vi "SVFA Unit Conversion (XY) (N Ch - M Orders).vi"(0 "magnitudes":T1(array[cluster]) {"magnitude" format="%.2f"; "time/rev/rpm" format="%.2f"}, 1 "desired scaling":T8 {"dB reference (0: no change)" format="%.2f"}, 4 "magnitudes info in":T2[](array[typedef]) {"x-axis units" items=["Time (s)"=0, "Frequency-CB (Hz)"=1, "Frequency-CPB (Hz)"=1248, "Frequency-Arbitrary (Hz)"=2357, "Quefrency (s)"=2, "Revolutions (rev)"=3, "Order"=4, "Speed (RPM)"=11, "Speed (rad/s)"=21, "Index"=65535]; "weighting filter" items=["Linear", "A-weighting", "B-weighting", "C-weighting", "ITU-R 468-4", "Dolby", "CCITT", "C-message", "Wb", "Wc", "Wd", "We", "Wf", "Wh", "Wj", "Wk", "Wm", "AES17 20 kHz lowpass", "AES17 40 kHz lowpass", "AES17 20 kHz highpass", "AES17 40 kHz highpass"]; "dB reference [EU]" format="%.2f"; "engineering units" items=["custom..."=0, "V"=1, "A"=21, "C"=30, "pC"=31, "s"=32, "-"=29, "Pa"=2, "N"=20, "g"=3, "m/s^2"=4, "m/s"=5, "m"=6, "mm/s"=12, "mm"=13, "micron/s"=14, "micron"=15, "in/s^2"=7, "in/s"=8, "in"=9, "mil/s"=10, "mil"=11, "rad/s^2"=16, "rad/s"=17, "rad"=18, "deg/s^2"=26, "deg/s"=27, "deg"=28, "RPM"=22, "cycle/s^2"=23, "Hz"=24, "cycle"=25, "strain"=19]; "spectral info"."window" items=["None "=0, "Hanning"=1, "Hamming"=2, "Blackman-Harris"=3, "Exact Blackman"=4, "Blackman"=5, "Flat Top"=6, "4 Term B-Harris "=7, "7 Term B-Harris"=8, "Low Sidelobe"=9, "Force - Exponential"=10, "Gaussian"=62]}, 5 "error in (no error)":errorcluster) -> (14 "converted magnitudes":T1(array[cluster]) {"magnitude" format="%.2f"; "time/rev/rpm" format="%.2f"}, 15 "unit labels":string[](array[string]), 18 "magnitudes info out":T2[](array[typedef]) {"x-axis units" items=["Time (s)"=0, "Frequency-CB (Hz)"=1, "Frequency-CPB (Hz)"=1248, "Frequency-Arbitrary (Hz)"=2357, "Quefrency (s)"=2, "Revolutions (rev)"=3, "Order"=4, "Speed (RPM)"=11, "Speed (rad/s)"=21, "Index"=65535]; "weighting filter" items=["Linear", "A-weighting", "B-weighting", "C-weighting", "ITU-R 468-4", "Dolby", "CCITT", "C-message", "Wb", "Wc", "Wd", "We", "Wf", "Wh", "Wj", "Wk", "Wm", "AES17 20 kHz lowpass", "AES17 40 kHz lowpass", "AES17 20 kHz highpass", "AES17 40 kHz highpass"]; "dB reference [EU]" format="%.2f"; "engineering units" items=["custom..."=0, "V"=1, "A"=21, "C"=30, "pC"=31, "s"=32, "-"=29, "Pa"=2, "N"=20, "g"=3, "m/s^2"=4, "m/s"=5, "m"=6, "mm/s"=12, "mm"=13, "micron/s"=14, "micron"=15, "in/s^2"=7, "in/s"=8, "in"=9, "mil/s"=10, "mil"=11, "rad/s^2"=16, "rad/s"=17, "rad"=18, "deg/s^2"=26, "deg/s"=27, "deg"=28, "RPM"=22, "cycle/s^2"=23, "Hz"=24, "cycle"=25, "strain"=19]; "spectral info"."window" items=["None "=0, "Hanning"=1, "Hamming"=2, "Blackman-Harris"=3, "Exact Blackman"=4, "Blackman"=5, "Flat Top"=6, "4 Term B-Harris "=7, "7 Term B-Harris"=8, "Low Sidelobe"=9, "Force - Exponential"=10, "Gaussian"=62]}, 19 "error out":errorcluster)   [LabVIEW 2017]
doc: "Converts between dB/linear, magnitude/magnitude^2, rms/peak/peak-peak, spectrum/spectral density, and dB ref1/dB ref2. Wire data to the <B>spectrum</B> input to determine the polymorphic instance to use or manually select the instance."
uses:
  <vilib>/addons/_NISVFA/_Shared subVIs/Controls/svc_Spectrum Info.ctl
  <vilib>/addons/_NISVFA/_Shared subVIs/Controls/svc_X-Axis Units.ctl
  <vilib>/addons/_NISVFA/_Shared subVIs/Controls/svc_Spectrum Type.ctl
  <vilib>/addons/_NISVFA/_Shared subVIs/Controls/svc_Engineering Units Text Ring.ctl
  <vilib>/addons/_NISVFA/_Shared subVIs/Controls/svc_Weighting Filter Text Ring.ctl
  <vilib>/addons/_NISVFA/_Shared subVIs/Controls/svc_Complimentary Spectrum Units.ctl
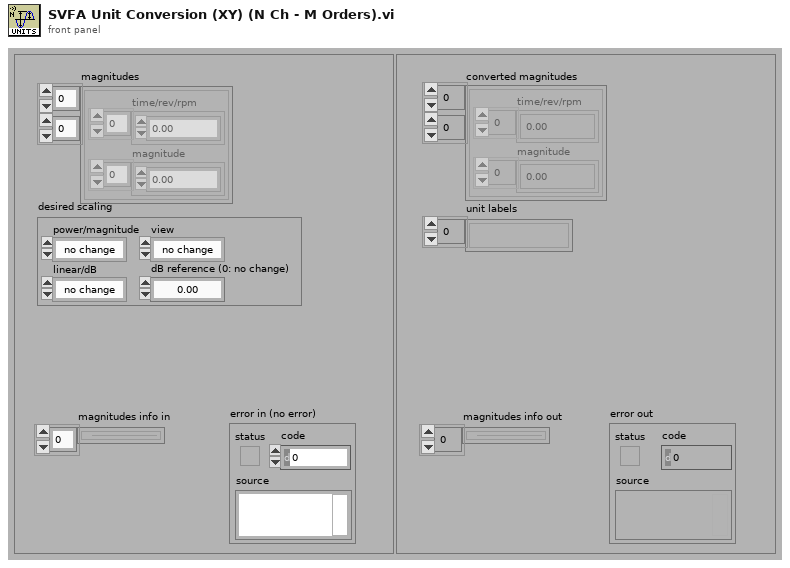
[diagram p1: front panel]
types:
  T1 = cluster{"time/rev/rpm":dbl[], "magnitude":dbl[]}[][]
  T2 = typedef "svc_Spectrum Info.ctl" = cluster{"channel name":string, "description":string, "x-axis units":T3, "spectral info":cluster{"spectrum type":T4, "linear/dB":enum16{"linear", "dB"}, "window":u16, "window size":i32, "FFT size":i32}, "engineering units":T5, "custom label":string, "dB reference [EU]":dbl, "peak units":enum16{"rms", "peak", "peak-peak"}, "weighting filter":T6, "spectral density?":bool, "unit label":string, "spectrum skewed?":bool, "complimentary spectrum units":T7}
  T3 = typedef "svc_X-Axis Units.ctl" = u16
  T4 = typedef "svc_Spectrum Type.ctl" = enum16{"FFT Spectrum [complex]", "Amplitude [Magnitude]", "Power [Magnitude^2]", "Cross Spectrum [complex]", "Frequency Response [Complex]"}
  T5 = typedef "svc_Engineering Units Text Ring.ctl" = u16
  T6 = typedef "svc_Weighting Filter Text Ring.ctl" = u16
  T7 = typedef "svc_Complimentary Spectrum Units.ctl" = enum16{"none", "radians", "degrees", "cycles", "imaginary"}
  T8 = cluster{"linear/dB":enum16{"no change", "linear", "dB"}, "dB reference (0: no change)":dbl, "power/magnitude":enum16{"no change", "power", "magnitude"}, "view":enum16{"no change", "rms", "peak", "peak-peak"}}
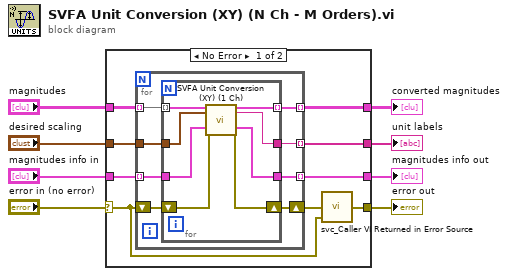
[diagram p0: block diagram]
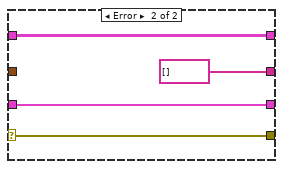
[diagram p2: hidden frame]
diagram:
  n1 = case shown="No Error" "error in (no error)" {
    selector: "error in (no error)" -> [w9 w37]
    tunnel: "magnitudes info in" -> [w17 w36]
    tunnel: "magnitudes" -> [w16 w35]
    tunnel: "desired scaling" -> [w15 _]
    tunnel: [w10 w37] -> w5
    tunnel: [w13 w35] -> w4
    tunnel: [w12 w36] -> w3
    tunnel: [w11 string[] []] -> w2
    frame No Error {
      n2 = for {
        tunnel: [w25] -> w13 mode=indexing
        shift-right: [w24] -> w14
        shift-left: w9 -> [w23]
        tunnel: w17 -> [w20] mode=indexing
        tunnel: w16 -> [w22] mode=indexing
        tunnel: w15 -> [w21]
        tunnel: [w19] -> w12 mode=indexing
        tunnel: [w18] -> w11 mode=indexing
        n3 = for {
          tunnel: [w33] -> w25 mode=indexing
          tunnel: w22 -> [w30] mode=indexing
          tunnel: w21 -> [w29]
          tunnel: w20 -> [w28]
          tunnel: [w27] -> w19
          tunnel: [w26] -> w18
          shift-right: [w32] -> w24
          shift-left: w23 -> [w31]
          n4 = call <vilib>:"SVFA Unit Conversion (XY) (1 Ch).vi"("magnitudes"=w30, "desired scaling"=w29, "magnitude info in"=w28, "error in (no error)"=w31) -> ("converted magnitudes"=w33:cluster{"time/rev/rpm":dbl[], "magnitude":dbl[]}, "unit label"=w26:string, "magnitude info out"=w27:T2, "error out"=w32:errorcluster)  [unwired: 12 in]
        }
      }
      n5 = call <vilib>:"svc_Caller VI Returned in Error Source.vi"("warning input to caller"=w9, "error in (no error)"=w14) -> ("error out"=w10:errorcluster)  [unwired: 3 in]
    }
    frame Error {
    }
  }
  "error out" <- w5
  "magnitudes info out" <- w3
  "converted magnitudes" <- w4
  "unit labels" <- w2
